vi "NI_SignalList.vi"(11 "XNET Database":refnum<k21>="HA_FJ20220115") -> (3 "SignalList":refnum<k21>[](array[refnum]))   [LabVIEW 2019]
uses:
  <resource>/objmgr/xnet.rc
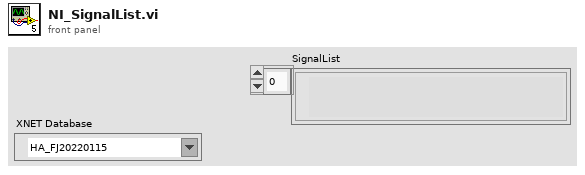
[diagram p1: front panel]
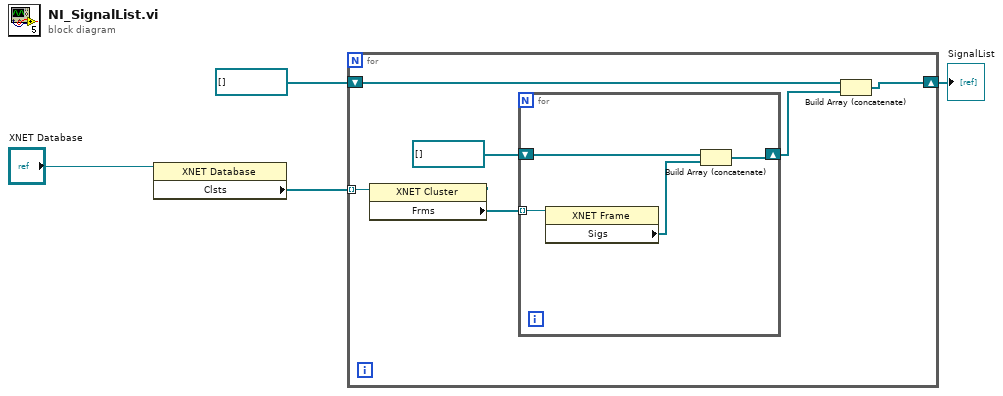
[diagram p0: block diagram]
diagram:
  n1 = property class="XNET Database"(reference="XNET Database") -> ("Clsts"=w3:refnum<k21>[])  [unwired: 1 in, 2 out]
  n2 = for {
    tunnel: w3 -> [w10] mode=indexing
    shift-right: [w5] -> w1
    shift-left: refnum<k21>[] [] -> [w7]
    n3 = property class="XNET Cluster"(reference=w10) -> ("Frms"=w9:refnum<k21>[])  [unwired: 1 in, 2 out]
    n4 = for {
      tunnel: w9 -> [w14] mode=indexing
      shift-right: [w11] -> w6
      shift-left: refnum<k21>[] [] -> [w13]
      n5 = property class="XNET Frame"(reference=w14) -> ("Sigs"=w12:refnum<k21>[])  [unwired: 1 in, 2 out]
      n6 = Build Array (concatenate)(w13, w12) -> (w11:refnum<k21>[])
    }
    n7 = Build Array (concatenate)(w7, w6) -> (w5:refnum<k21>[])
  }
  "SignalList" <- w1
